vi "LabviewPython_reset.vi"(6 "frdOmr_":bool, 7 "reset_":bool, 8 "movie L":dbl, 9 "movie R":dbl, 10 "forward_":dbl, 11 "yaw_":dbl) -> (0 "vreFps":dbl, 1 "HA_":dbl, 2 "y_":dbl, 3 "x_":dbl)   [LabVIEW 2012]
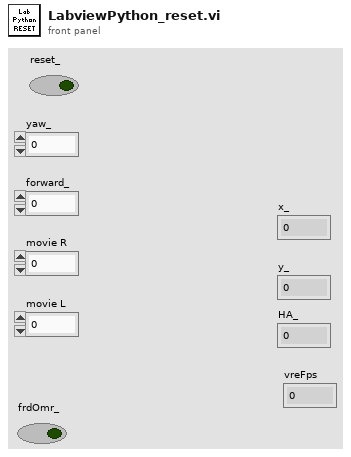
[diagram p1: front panel]
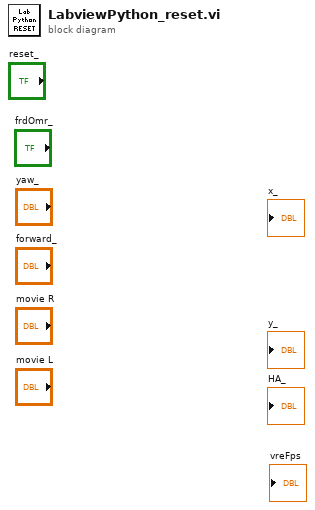
[diagram p0: block diagram]
diagram:
